vi "Stop Acquisition.vi"(8 "error in (no error)":errorcluster, 11 "Hardware Resources in":T1={"AI"={"DAQmx Channel"="", "Max Input"=0.0, "Min Input"=0.0, "Sample Rate"=0.0, "DAQmx Task"="", "shunt resistor location"=-1, "external shunt resistor value"=249.0}, "AO"={"DAQmx Channel"="", "Max Output"=0.0, "Min Output"=0.0, "Sample Rate"=0.0, "DAQmx Task"=""}, "DO"={"DAQmx Channel"="", "Sample Rate"=0.0, "DAQmx Task"=""}, "DI"={"DAQmx Channel"="", "Sample Rate"=0.0, "DAQmx Task"=""}, "TC"={"DAQmx Channel"="", "Max Inout"=0.0, "Min Input"=0.0, "Sample Rate"=0.0, "DAQmx Task"="", "resistance configuration"=4, "r0"=100.0, "current excitation value"=0.0025, "current excitation source"=10167, "rtd type"=12481}} {"TC"."rtd type" items=["Pt3750"=12481, "Pt3851"=10071, "Pt3911"=12482, "Pt3916"=10069, "Pt3920"=10053, "Pt3928"=12483, "Custom"=10137]; "TC"."current excitation source" items=["Internal"=10200, "External"=10167, "None"=10230]; "TC"."resistance configuration" items=["2-Wire"=2, "3-Wire"=3, "4-Wire"=4]; "AI"."shunt resistor location" items=["default"=-1, "RSE"=10083, "NRSE"=10078, "Differential"=10106, "Pseudodifferential"=12529]}) -> (0 "error out":errorcluster)   [LabVIEW 2024, in "Acquisition.lvlib"]
doc: "Stops the acquisition."
uses:
  Acquisition.lvlib
  Hardware Configuration.ctl
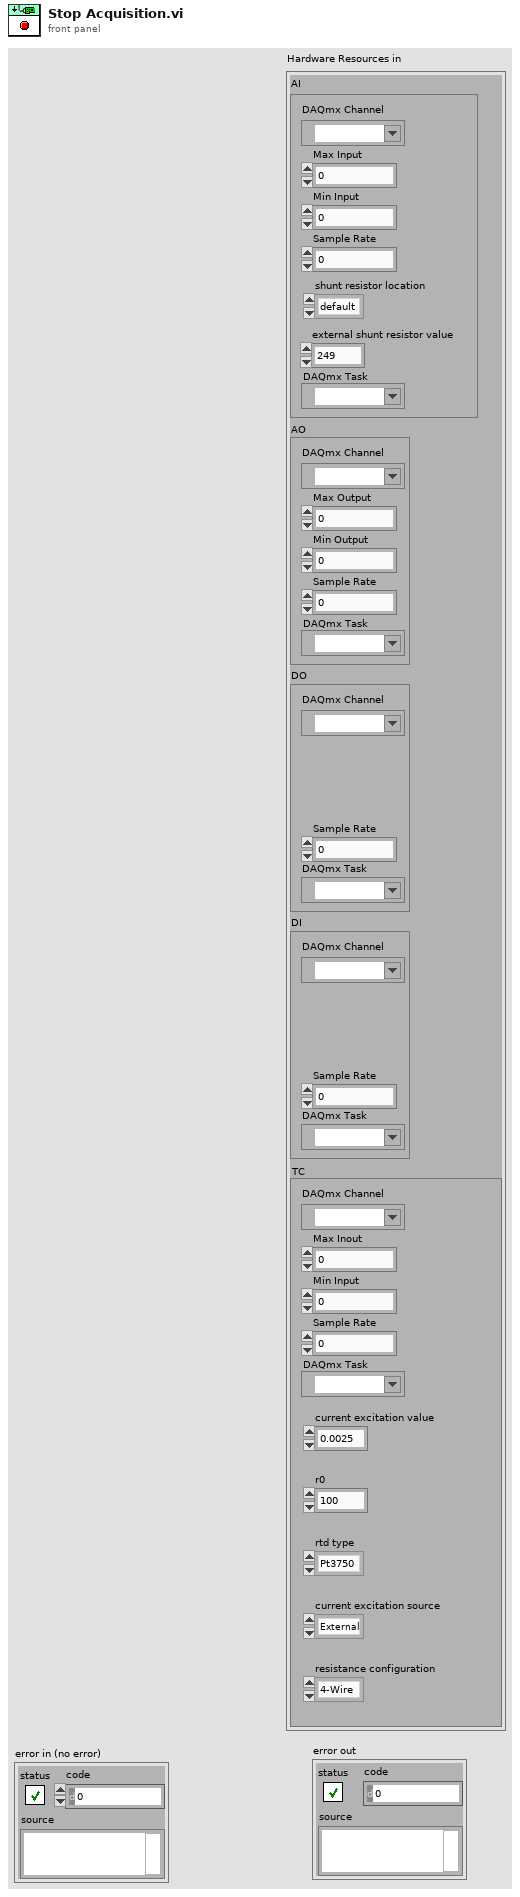
[diagram p1: front panel]
types:
  T1 = typedef "Acquisition.lvlib/Hardware Configuration.ctl" = cluster{"AI":cluster{"DAQmx Channel":tag, "Max Input":dbl, "Min Input":dbl, "Sample Rate":dbl, "DAQmx Task":refnum<k21>, "shunt resistor location":i32, "external shunt resistor value":dbl}, "AO":cluster{"DAQmx Channel":tag, "Max Output":dbl, "Min Output":dbl, "Sample Rate":dbl, "DAQmx Task":refnum<k21>}, "DO":cluster{"DAQmx Channel":tag, "Sample Rate":dbl, "DAQmx Task":refnum<k21>}, "DI":cluster{"DAQmx Channel":tag, "Sample Rate":dbl, "DAQmx Task":refnum<k21>}, "TC":cluster{"DAQmx Channel":tag, "Max Inout":dbl, "Min Input":dbl, "Sample Rate":dbl, "DAQmx Task":refnum<k21>, "resistance configuration":i32, "r0":dbl, "current excitation value":dbl, "current excitation source":i32, "rtd type":i32}}
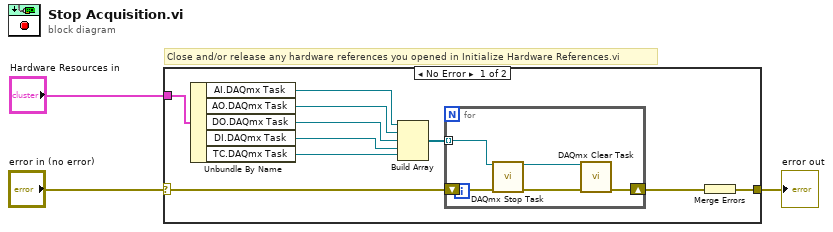
[diagram p0: block diagram]
diagram:
  # "Close and/or release any hardware references you opened in Initialize Hardware References.vi"
  n1 = case shown="No Error" "error in (no error)" {
    selector: "error in (no error)" -> [w12 w19]
    tunnel: [w13 w19] -> w2
    tunnel: "Hardware Resources in" -> [w10 _]
    frame No Error {
      n2 = Unbundle By Name(w10) -> ("AI.DAQmx Task"=w5:refnum<k21>, "AO.DAQmx Task"=w6:refnum<k21>, "DO.DAQmx Task"=w7:refnum<k21>, "DI.DAQmx Task"=w8:refnum<k21>, "TC.DAQmx Task"=w9:refnum<k21>)
      n3 = Build Array(w5, w6, w7, w8, w9) -> (w4:refnum<k21>[])
      n4 = for {
        shift-right: [w15] -> w11
        shift-left: w12 -> [w18]
        tunnel: w4 -> [w14] mode=indexing
        n5 = call <vilib>:"DAQmx Stop Task.vi"("task/channels in"=w14, "error in"=w18) -> ("task out"=w17:refnum<k21>, "error out"=w16:errorcluster)  [unwired: 12 in]
        n6 = call <vilib>:"DAQmx Clear Task.vi"("task in"=w17, "error in"=w16) -> ("error out"=w15:errorcluster)  [unwired: 13 in]
      }
      n7 = Merge Errors(w11) -> (w13:errorcluster)
    }
    frame Error {
    }
  }
  "error out" <- w2
